vi "ReadInitParameters.vi"(8 "error in (no error)":errorcluster, 11 "INI Filepath":path) -> (0 "error out":errorcluster, 3 "Init Parameters":T1)   [LabVIEW 2020, in "StashRoyale.lvclass"]
uses:
  StashRoyale.lvclass
  <vilib>/Utility/config.llb/NI_LVConfig.lvlib
  InitParameters.ctl
  <vilib>/Utility/config.llb/Read Key (String).vi
  <vilib>/Utility/config.llb/Read Key (Path).vi
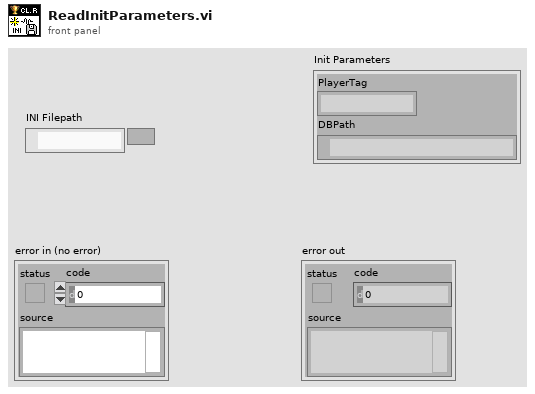
[diagram p1: front panel]
types:
  T1 = typedef "InitParameters.ctl" = cluster{"PlayerTag":string, "DBPath":path}
  T2 = typedef "NI_LVConfig.lvlib/Config Data RefNum.ctl" = refnum<k1>
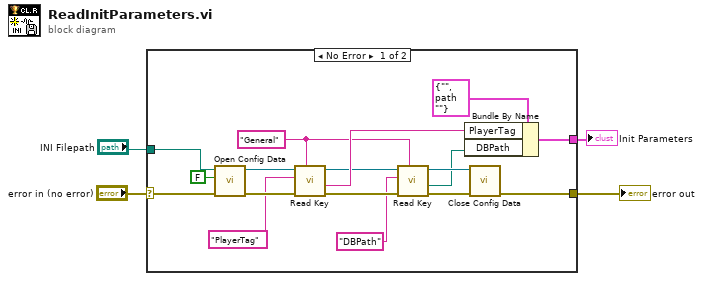
[diagram p0: block diagram]
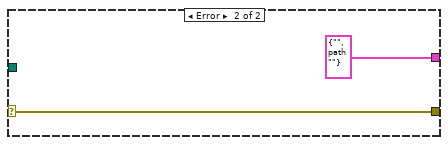
[diagram p2: hidden frame]
diagram:
  n1 = case shown="No Error" "error in (no error)" {
    selector: "error in (no error)" -> [w16 w23]
    tunnel: "INI Filepath" -> [w21 _]
    tunnel: [w15 w23] -> w2
    tunnel: [w12 T1 {"PlayerTag"="", "DBPath"=path ""} ("Init Parameters")] -> w1
    frame No Error {
      w11 = "General" ("section")
      n2 = call <vilib>:"Open Config Data.vi"("error in (no error)"=w16, "create file if necessary (T)"=FALSE, "configuration file path"=w21) -> ("error out"=w18:errorcluster, "refnum"=w19:T2)  [unwired: 6 in, 1 out]
      n3 = call-poly <vilib>:"Read Key.vi"("section"=w11, "error in (no error)"=w18, "key"="PlayerTag", "refnum"=w19) -> ("error out"=w9:errorcluster, "value"=w13:string, "refnum out"=w10:T2)  [unwired: 4 in, 1 out]
      n4 = call-poly <vilib>:"Read Key.vi"("section"=w11, "error in (no error)"=w9, "key"="DBPath", "refnum"=w10) -> ("error out"=w7:errorcluster, "value"=w5:path, "refnum out"=w6:T2)  [unwired: 4 in, 1 out]
      n5 = Bundle By Name(cluster=T1 {"PlayerTag"="", "DBPath"=path ""} ("Init Parameters"), "PlayerTag"=w13, "DBPath"=w5) -> (w12:T1)
      n6 = call <vilib>:"Close Config Data.vi"("error in (no error)"=w7, "refnum"=w6) -> ("error out"=w15:errorcluster)  [unwired: 8 in, 1 out]
    }
    frame Error {
    }
  }
  "Init Parameters" <- w1
  "error out" <- w2
